vi "MakeChannel.vi"(4 "Power Line\nConfigurations":T2[](array[typedef]) {"Max Current [A]" format="%#_13g"; "Min Current [A]" format="%#_13g"; "Shunt Resistor [Ohm]" format="%#_13g"}, 6 "Power Line\nQuantity":T1, 8 "Input Error":errorcluster, 9 "Power Line\nEnable":bool[](array[boolean])=[TRUE], 10 "Power Line\nChannels":tag[](array[tag]), 11 "Input Task":refnum<k21>) -> (0 "Output Error":errorcluster, 3 "Output Task":refnum<k21>)   [LabVIEW 2020]
uses:
  PowerLineConfig.ctl
  PowerLineQuantity.ctl
  <vilib>/DAQmx/create/channels.llb/DAQmx Create Channel (AI-Current-Basic).vi
  <vilib>/DAQmx/create/channels.llb/DAQmx Create Channel (AI-Voltage-Basic).vi
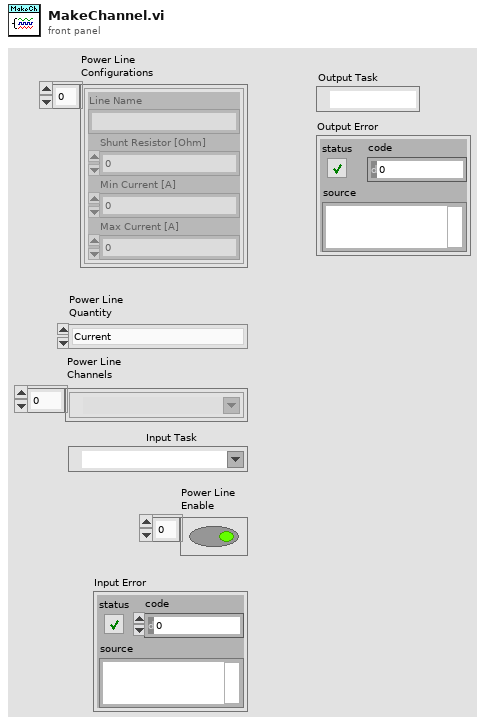
[diagram p1: front panel]
types:
  T1 = typedef "PowerLineQuantity.ctl" = enum16{"Current", "Voltage"}
  T2 = typedef "PowerLineConfig.ctl" = cluster{"Line Name":string, "Shunt Resistor [Ohm]":dbl, "Min Current [A]":dbl, "Max Current [A]":dbl}
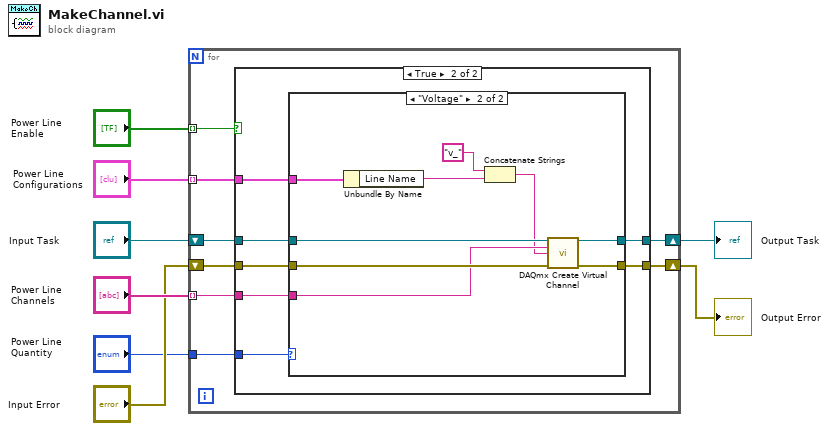
[diagram p0: block diagram]
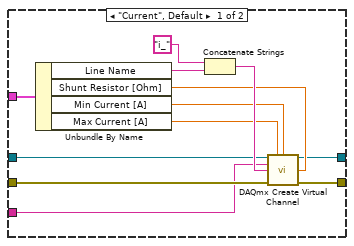
[diagram p3: hidden frame]
diagram:
  n1 = for {
    tunnel: "Power Line\nEnable" -> [w10] mode=indexing
    tunnel: "Power Line\nChannels" -> [w11] mode=indexing
    tunnel: "Power Line\nConfigurations" -> [w9] mode=indexing
    shift-right: [w14] -> w2
    shift-left: "Input Task" -> [w12]
    shift-right: [w16] -> w1
    shift-left: "Input Error" -> [w13]
    tunnel: "Power Line\nQuantity" -> [w15]
    n2 = case shown="True" w10 {
      tunnel: [w18 w25] -> w16
      tunnel: w15 -> [_ w24]
      tunnel: [w17 w23] -> w14
      tunnel: w13 -> [w18 w22]
      tunnel: w12 -> [w17 w21]
      tunnel: w11 -> [_ w20]
      tunnel: w9 -> [_ w19]
      frame False {
      }
      frame True {
        n3 = case shown="\"Voltage\"" w24 {
          tunnel: [w26 w38] -> w25
          tunnel: [w27 w39] -> w23
          tunnel: w22 -> [w30 w46]
          tunnel: w21 -> [w31 w45]
          tunnel: w20 -> [w29 w44]
          tunnel: w19 -> [w28 w43]
          frame "Current", Default {
            n4 = Unbundle By Name(w28) -> ("Line Name"=w36:string, "Shunt Resistor [Ohm]"=w34:dbl, "Min Current [A]"=w33:dbl, "Max Current [A]"=w32:dbl)
            n5 = Concatenate Strings("i_", w36) -> (w37:string)
            n6 = call-poly <vilib>:"DAQmx Create Virtual Channel.vi"("task in"=w31, "maximum value"=w32, "minimum value"=w33, "physical channels"=w29, "name to assign"=w37, "external shunt resistor value"=w34, "error in"=w30) -> ("task out"=w27:refnum<k21>, "error out"=w26:errorcluster)  [unwired: 7 in]
          }
          frame "Voltage" {
            n7 = Unbundle By Name(w43) -> ("Line Name"=w41:string)
            n8 = Concatenate Strings("v_", w41) -> (w40:string)
            n9 = call-poly <vilib>:"DAQmx Create Virtual Channel.vi"("task in"=w45, "physical channels"=w44, "name to assign"=w40, "error in"=w46) -> ("task out"=w39:refnum<k21>, "error out"=w38:errorcluster)  [unwired: 10 in]
          }
        }
      }
    }
  }
  "Output Task" <- w2
  "Output Error" <- w1
